vi "NIMS_NS_iir_lpnormconstr.vi"(5 "Function name":string, 6 "Line number":i32, 7 "Number of outputs requested":i32, 8 "error in (no error)":errorcluster, 11 "[A]":variant[](array[variant])) -> (0 "error out":errorcluster, 3 "[funct(A)]":variant[](array[variant]))   [LabVIEW 2017]
uses:
  <vilib>/imath/engines/lvmath/Functions/Error Handling/error.ctl
  <instcachedir>/0/NIMS_RunTimeType_From StrictType (excl LVString)_1019F277F0A747EDBCA0F6C52CA54500.lvgen/NIMS_RunTimeType_From StrictType (excl LVString)_1019F277F0A747EDBCA0F6C52CA54500_000.vi
  <instcachedir>/0/NIMS_Get Scalar_w Error_1987D997E87247DDAC16EA23A5E9E4FC.lvgen/NIMS_Get Scalar_w Error_1987D997E87247DDAC16EA23A5E9E4FC_000.vi
  <instcachedir>/0/NIMS_Complex To Real_BE01396FDE034E8E94CEBBA1E368668D.lvgen/NIMS_Complex To Real_BE01396FDE034E8E94CEBBA1E368668D_000.vi
  <instcachedir>/0/NIMS_Get Any Vector_w Error - Matrix_9FDB8FBE264C42EDBC8FF9BA66C3EF33.lvgen/NIMS_Get Any Vector_w Error - Matrix_9FDB8FBE264C42EDBC8FF9BA66C3EF33_001.vi
  <instcachedir>/0/NIMS_Get Scalar_w Error_1987D997E87247DDAC16EA23A5E9E4FC.lvgen/NIMS_Get Scalar_w Error_1987D997E87247DDAC16EA23A5E9E4FC_003.vi
  <instcachedir>/0/NIMS_RunTimeType_To Numeric_1CBDAFC4EFAD4045A1DE52278D16738D.lvgen/NIMS_RunTimeType_To Numeric_1CBDAFC4EFAD4045A1DE52278D16738D_000.vi
  <vilib>/addons/Digital Filter Design/NI_DigFilter_MathScript.lvlib
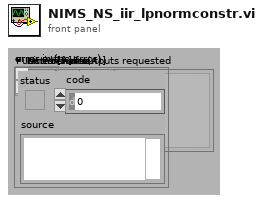
[diagram p1: front panel]
types:
  T1 = typedef "error.ctl" = enum16{"No Error", "Problem", "Input type must not be void", "Incorrect number of parameters", "Function not defined for non-numeric types", "An output variable of the user-defined function is undefined", "Function only defined for character arrays", "Function not defined for boolean, character, or single precision", "Function not defined for complex types", "Not a valid operation", "Inputs must be scalar", "Input matrices are not the same size", "Function only available on RT", "Input matrices must be nonnegative integers of the same type", "Arguments must be non-negative integers less than bitmax", "Number to complement must be less than 2^N", "Bit to get is outside range", "Bit to set is outside range", "Input must be real type ", "At least one parameter must be scalar", "Unable to display plug-in data on RT", "Function not defined for higher dimensional matrices", "Invalid attributes", "Wrong Type of Input Arguments", "Wrong Argument Option", "Invalid file identifier", "Indices must be real positive integers", "The variable is not a matrix data type.", "Number of elements must be the same for indices and values", "You cannot replace elements of a matrix with non-matrix data types.", "Cannot resize a 2D matrix with a linear index", "Unknown variable or symbol", "Indices out of range", "Empty matrix deletion can not be used with two indices", "Number of rows and columns must be the same for indices and values.", "Complex cannot be converted to Boolean", "Char cannot be converted to Boolean", "int64 cannot be converted to Boolean", "uint64 cannot be converted to Boolean", "You cannot convert a Boolean to a character.", "Incompatible input size in 3D surface function", "All rows must have the same number of columns", "Incompatible types", "Invalid matrix dimensions", "Dimension must be 1 or 2", "Base must be an integer between 2 and 36", "Invalid input", "Square matrix required", "Function 'timerstart' must be called before 'timerstop'", "Arguments must be positive real", "Step must not be zero", "Wrong number of input arguments", "Wrong number of output arguments", "Too many index arguments", "Input scalar must be >= 0", "Input scalar must be positive", "Input scalar must not be 0", "Input scalar must be in range [0,1]", "Can't use conditionally defined variable that's undefined", "Input must be a vector", "RT Exec Trace Toolkit not licensed", "Empty vector error", "All elements must be in domain [-1,1]", "All real elements of input vector must be >= 0", "All elements of input vector must be positive", "Values of input vectors are not compatible", "DAQmx not installed", "Input vector must be an increasing vector", "Dereferenced field does not exist within the struct", "A vector or matrix of structures must be indexed before it can be dereferenced", "Lenths of two input vectors are not compatible", "Invalid fieldname", "Empty matrix error", "Cannot use '.' on a type other than Struct", "Unused074", "Data type of the struct's field name is invalid", "Using . to dereference data that is not a struct", "Input struct contains invalid type ", "Size of input matrix is incompatible with input size", "Invalid format specifier", "Could not find field within struct", "Bad permutation array", "Mismatched fieldnames", "ode: User Function could not be opened", "ode: User Function signature does not meet ode requirements", "Unused085", "RunTime: MathScript could not be compiled", "Unknown function", "Only scalars and strings supported", "ode: User Function signature has incorrect number of inputs", "ode:User Function signature has incorrect number of outputs", "Range is too large", "End used without variable", "Function not available (RTE)", "Custom user error", "Arguments must be integers less than bitmax", "Shared library not found", "Header file not found", "Shared library already loaded", "Shared library not loaded", "Shared library function not found", "Shared library string return problem", "Problem calling shared library function", "Problem loading shared library from OS", "Problem parsing shared library header file", "Shared library incompatible types", "Shared library unsupported return type", "Shared library function not exported", "Shared library unsupported input type", "Problem unloading shared library from OS", "Function only available from UI", "Function specified in argument is missing", "An internal error has occurred", "Invalid object", "Invalid property", "Read-only property", "A break command has occurred", "A continue command has occurred", "A return command has occurred", "ode: times parameter invalid", "Function specified in argument has incorrect signature", "Function not found in file", "Reserved keyword cannot be defined as variable", "Reserved keyword cannot be defined as a function or script", "Arguments must be string literals", "Function not supported on this platform", "All columns must have the same number of rows", "Function ignored in RTE warning", "Cannot use : as a parameter that is not a variable", "Output can't be coerced to requested type", "Function not supported on current target", "Variable dependent on an unwired function input", "Unused132", "Unused133", "Unused134", "Unused135", "Unused136", "Unused137", "Unused138", "Unused139", "Global/Persistent must only take constants as arguments.", "Varargin must be last input in the function definition.", "Varargout must be last output in the function definition.", "Invalid output type. Cannot output a cell array of any type other than string.", "Invalid output type. Type is a dynamic struct.", "Invalid output type. Type is a struct that has a field whose type is not known until run-time", "Invalid output type. Type is a struct that has a field which is a plot object.", "MathScript parser DLL missing", "MathScript requires LabVIEW Full", "MathScript license is invalid or missing", "Varargout not supported except in assignments."}
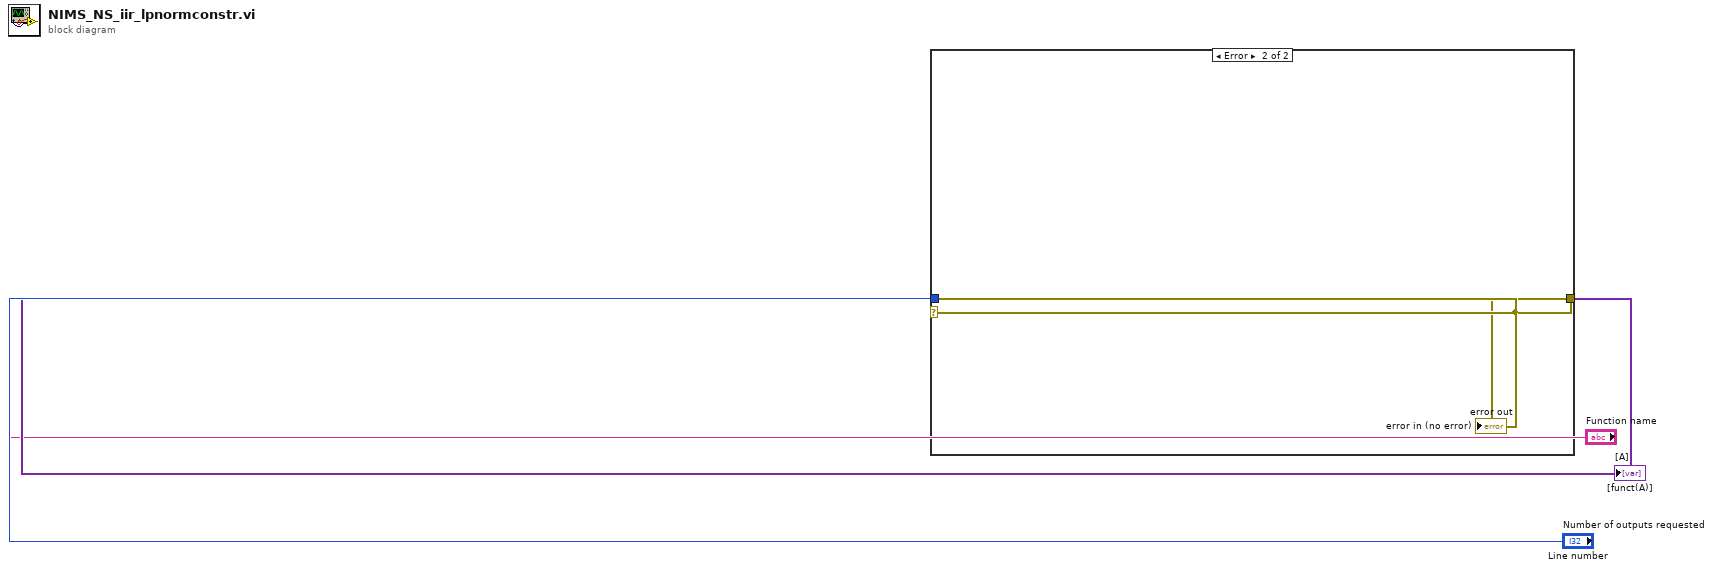
[diagram p0: block diagram]
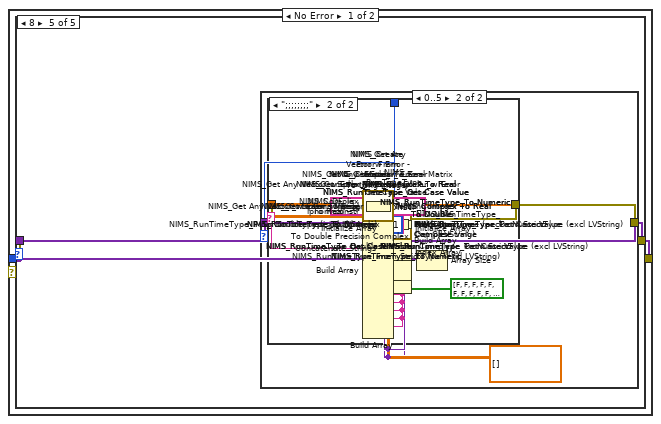
[diagram p2: hidden frame]
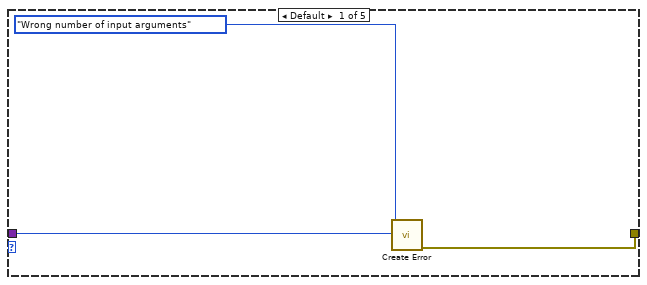
[diagram p3: hidden frame]
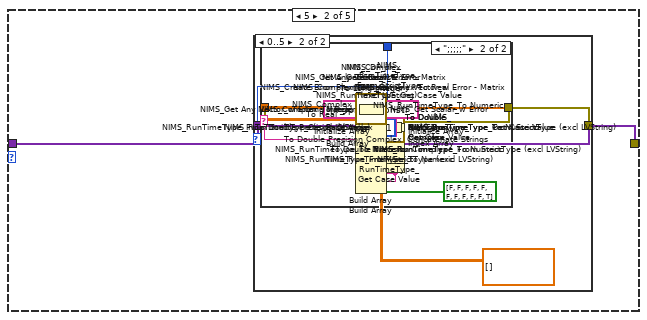
[diagram p4: hidden frame]
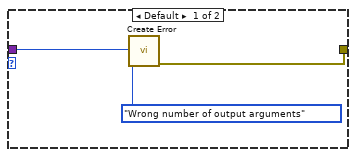
[diagram p5: hidden frame]
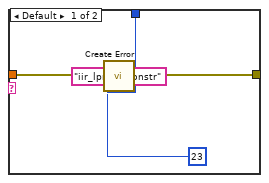
[diagram p6: hidden frame]
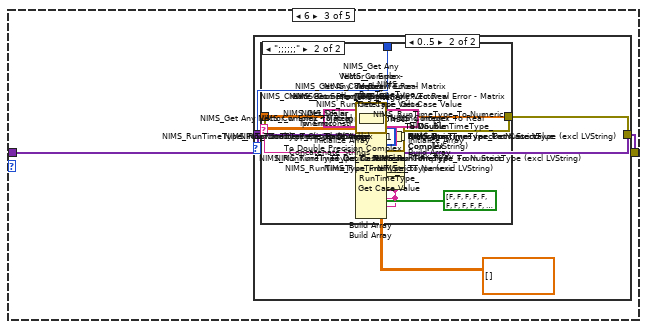
[diagram p7: hidden frame]
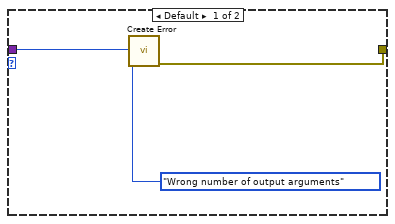
[diagram p8: hidden frame]
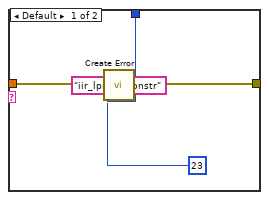
[diagram p9: hidden frame]
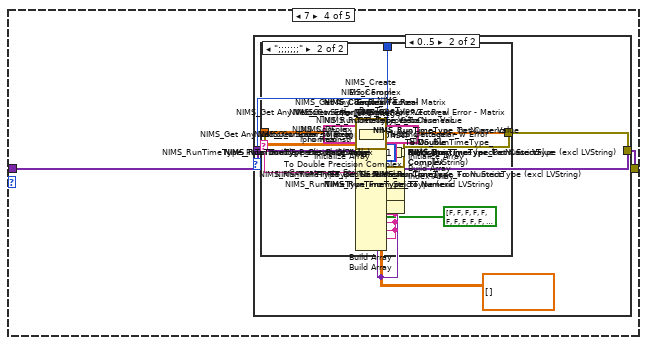
[diagram p10: hidden frame]
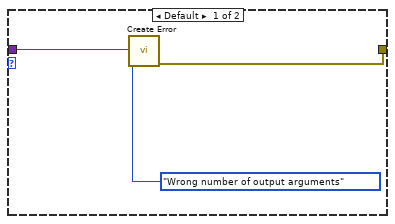
[diagram p11: hidden frame]
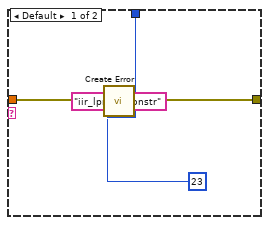
[diagram p12: hidden frame]
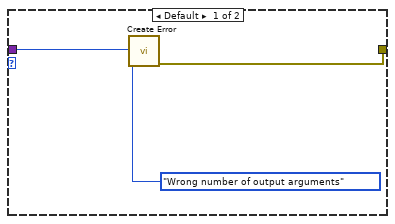
[diagram p13: hidden frame]
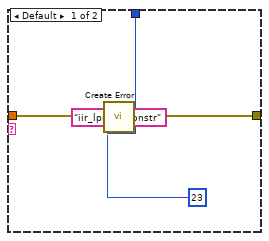
[diagram p14: hidden frame]
diagram:
  n1 = case shown="Error" "error in (no error)" {
    selector: "error in (no error)" -> [_ w516]
    tunnel: [w15 _] -> w4
    tunnel: [w14 w516] -> w3
    tunnel: "error in (no error)" -> [w13 _]
    tunnel: "Number of outputs requested" -> [w12 _]
    tunnel: "[A]" -> [w11 _]
    tunnel: "Function name" -> [w10 _]
    tunnel: "Line number" -> [w9 _]
    frame No Error {
      n2 = Array Size(array=w11) -> (size(s)=w8:i32)
      n3 = case shown="8" w8 {
        tunnel: [_ w27 w137 w256 w384] -> w15
        tunnel: w10 -> [w19 w24 w134 w253 w381]
        tunnel: w9 -> [w20 w25 w135 w254 w382]
        tunnel: w13 -> [w17 w23 w133 w252 w380]
        tunnel: [w16 w22 w132 w251 w379] -> w14
        tunnel: w12 -> [_ w21 w131 w250 w378]
        tunnel: w11 -> [_ w26 w136 w255 w383]
        frame Default {
          n4 = call <vilib>:"Create Error.vi"("Function name"=w19, "error in (no error)"=w17, "Error Enum"=error."Wrong number of input arguments", "Line number"=w20) -> ("error out"=w16:errorcluster)  [unwired: 6 in, 1 out]
        }
        frame 5 {
          n5 = case shown="0..5" w21 {
            tunnel: [_ w33] -> w27
            tunnel: w24 -> [w31 _]
            tunnel: w25 -> [w32 w83]
            tunnel: w23 -> [w29 w81]
            tunnel: [w28 w60] -> w22
            tunnel: w26 -> [_ w84]
            frame Default {
              n6 = call <vilib>:"Create Error.vi"("Function name"=w31, "error in (no error)"=w29, "Error Enum"=error."Wrong number of output arguments", "Line number"=w32) -> ("error out"=w28:errorcluster)  [unwired: 6 in, 1 out]
            }
            frame 0..5 {
              w42 = 1
              w50 = 1
              n7 = Index Array(array=w84) -> (element #1=w80:variant, element #2=w76:variant, element #3=w72:variant, element #4=w68:variant, element #5=w64:variant)  [unwired: 5 in]
              n8 = call <vilib>:"NIMS_RunTimeType_Get Case Value.vi"("Data In"=w64) -> ("Case Value"=w61:string)  [unwired: 9 in, 1 out]
              n9 = call-generic <vilib>:"NIMS_RunTimeType_To Numeric.vi"("DataType"=cdb[][] [], "Variant"=w64) -> ("data"=w62:cdb[][])  [unwired: 1 in]
              n10 = call <vilib>:"NIMS_RunTimeType_Get Case Value.vi"("Data In"=w68) -> ("Case Value"=w65:string)  [unwired: 9 in, 1 out]
              n11 = call-generic <vilib>:"NIMS_RunTimeType_To Numeric.vi"("DataType"=cdb[][] [], "Variant"=w68) -> ("data"=w66:cdb[][])  [unwired: 1 in]
              n12 = call <vilib>:"NIMS_RunTimeType_Get Case Value.vi"("Data In"=w72) -> ("Case Value"=w69:string)  [unwired: 9 in, 1 out]
              n13 = call-generic <vilib>:"NIMS_RunTimeType_To Numeric.vi"("DataType"=cdb[][] [], "Variant"=w72) -> ("data"=w70:cdb[][])  [unwired: 1 in]
              n14 = call <vilib>:"NIMS_RunTimeType_Get Case Value.vi"("Data In"=w76) -> ("Case Value"=w73:string)  [unwired: 9 in, 1 out]
              n15 = call-generic <vilib>:"NIMS_RunTimeType_To Numeric.vi"("DataType"=cdb[][] [], "Variant"=w76) -> ("data"=w74:cdb[][])  [unwired: 1 in]
              n16 = call <vilib>:"NIMS_RunTimeType_Get Case Value.vi"("Data In"=w80) -> ("Case Value"=w77:string)  [unwired: 9 in, 1 out]
              n17 = call-generic <vilib>:"NIMS_RunTimeType_To Numeric.vi"("DataType"=cdb[][] [], "Variant"=w80) -> ("data"=w78:cdb[][])  [unwired: 1 in]
              n18 = Concatenate Strings(w77, w73, w69, w65, w61) -> (w82:string)
              n19 = case shown="\";;;;;\"" w82 {
                tunnel: w81 -> [w86 w99]
                tunnel: [_ w94] -> w59
                tunnel: [_ w93] -> w55
                tunnel: [_ w92] -> w51
                tunnel: [_ w91] -> w46
                tunnel: [_ w90] -> w43
                tunnel: [w85 w95] -> w60
                tunnel: w78 -> [_ w129]
                tunnel: w74 -> [_ w125]
                tunnel: w70 -> [_ w121]
                tunnel: w66 -> [_ w118]
                tunnel: w62 -> [_ w115]
                tunnel: w83 -> [w89 w102]
                frame Default {
                  n20 = call <vilib>:"Create Error.vi"("Function name"="iir_lpnormconstr", "error in (no error)"=w86, "Error Enum"=23, "Line number"=w89) -> ("error out"=w85:errorcluster)  [unwired: 6 in, 1 out]
                }
                frame ";;;;;" {
                  w97 = "iir_lpnormconstr"
                  n21 = call-generic <vilib>:"NIMS_Complex To Real.vi"("A"=w115) -> ("Error Enum"=w105:T1, "Real(A)"=w114:dbl[][])  [unwired: 8 in, 1 out]
                  n22 = call-generic <vilib>:"NIMS_Get Any Vector_w Error - Matrix.vi"("A"=w114) -> ("Error Enum"=w104:T1, "Vector"=w116:dbl[])  [unwired: 8 in, 1 out]
                  n23 = call-generic <vilib>:"NIMS_Complex To Real.vi"("A"=w118) -> ("Error Enum"=w107:T1, "Real(A)"=w117:dbl[][])  [unwired: 8 in, 1 out]
                  n24 = call-generic <vilib>:"NIMS_Get Any Vector_w Error - Matrix.vi"("A"=w117) -> ("Error Enum"=w106:T1, "Vector"=w119:dbl[])  [unwired: 8 in, 1 out]
                  n25 = call-generic <vilib>:"NIMS_Complex To Real.vi"("A"=w121) -> ("Error Enum"=w109:T1, "Real(A)"=w120:dbl[][])  [unwired: 8 in, 1 out]
                  n26 = call-generic <vilib>:"NIMS_Get Any Vector_w Error - Matrix.vi"("A"=w120) -> ("Error Enum"=w108:T1, "Vector"=w122:dbl[])  [unwired: 8 in, 1 out]
                  n27 = call-generic <vilib>:"NIMS_Complex To Real.vi"("A"=w125) -> ("Error Enum"=w111:T1, "Real(A)"=w124:dbl[][])  [unwired: 8 in, 1 out]
                  n28 = To Long Integer(number=w124) -> (32bit integer=w123:i32[][])
                  n29 = call-generic <vilib>:"NIMS_Get Scalar_w Error.vi"("A"=w123) -> ("Error Enum"=w110:T1, "Scalar"=w126:i32)  [unwired: 8 in, 1 out]
                  n30 = call-generic <vilib>:"NIMS_Complex To Real.vi"("A"=w129) -> ("Error Enum"=w113:T1, "Real(A)"=w128:dbl[][])  [unwired: 8 in, 1 out]
                  n31 = To Long Integer(number=w128) -> (32bit integer=w127:i32[][])
                  n32 = call-generic <vilib>:"NIMS_Get Scalar_w Error.vi"("A"=w127) -> ("Error Enum"=w112:T1, "Scalar"=w130:i32)  [unwired: 8 in, 1 out]
                  n33 = call <vilib>:"NIMS_DF_iir_lpnormconstr.vi"("n"=w130, "e"=w119, "d"=w126, "f"=w122, "mag"=w116) -> ("b"=w94:dbl[], "a"=w93:dbl[], "err"=w92:dbl, "SOS"=w91:dbl[][], "error"=w103:i32, "gain"=w90:dbl)  [unwired: 5 in]
                  n34 = Build Array(w97, w97, w97, w97, w97, w97, w97, w97, w97, w97, "iir_lpnormconstr") -> (w100:string[])
                  n35 = Build Array(w113, w112, w111, w110, w109, w108, w107, w106, w105, w104, w103) -> (w101:i32[])
                  n36 = call <vilib>:"NIMS_Create Error From Enums.vi"("Error Code"=bool[] [FALSE, FALSE, FALSE, FALSE, FALSE, FALSE, FALSE, FALSE, FALSE, FALSE, TRUE], "error in (no error)"=w99, "Line no"=w102, "Error Enums"=w101, "Function names"=w100) -> ("error out"=w95:errorcluster)  [unwired: 6 in]
                }
              }
              n37 = To Double Precision Complex(1:w46) -> (0:w45:cdb[][])
              n38 = call-generic <vilib>:"NIMS_RunTimeType_From StrictType (excl LVString).vi"("Plug-In Name"="", "Data In"=w45) -> ("Data Out"=w35:variant)  [unwired: 2 in]
              n39 = Initialize Array(w43, w42, w42) -> (w41:dbl[][])
              n40 = To Double Precision Complex(1:w41) -> (0:w40:cdb[][])
              n41 = call-generic <vilib>:"NIMS_RunTimeType_From StrictType (excl LVString).vi"("Plug-In Name"="", "Data In"=w40) -> ("Data Out"=w34:variant)  [unwired: 2 in]
              n42 = Initialize Array(w51, w50, w50) -> (w49:dbl[][])
              n43 = To Double Precision Complex(1:w49) -> (0:w48:cdb[][])
              n44 = call-generic <vilib>:"NIMS_RunTimeType_From StrictType (excl LVString).vi"("Plug-In Name"="", "Data In"=w48) -> ("Data Out"=w36:variant)  [unwired: 2 in]
              n45 = Build Array(w55) -> (w54:dbl[][])
              n46 = To Double Precision Complex(1:w54) -> (0:w53:cdb[][])
              n47 = call-generic <vilib>:"NIMS_RunTimeType_From StrictType (excl LVString).vi"("Plug-In Name"="", "Data In"=w53) -> ("Data Out"=w37:variant)  [unwired: 2 in]
              n48 = Build Array(w59) -> (w58:dbl[][])
              n49 = To Double Precision Complex(1:w58) -> (0:w57:cdb[][])
              n50 = call-generic <vilib>:"NIMS_RunTimeType_From StrictType (excl LVString).vi"("Plug-In Name"="", "Data In"=w57) -> ("Data Out"=w38:variant)  [unwired: 2 in]
              n51 = Build Array(w38, w37, w36, w35, w34) -> (w33:variant[])
            }
          }
        }
        frame 6 {
          n52 = case shown="0..5" w131 {
            tunnel: [_ w143] -> w137
            tunnel: w134 -> [w141 _]
            tunnel: w135 -> [w142 w197]
            tunnel: w133 -> [w139 w195]
            tunnel: [w138 w170] -> w132
            tunnel: w136 -> [_ w198]
            frame Default {
              n53 = call <vilib>:"Create Error.vi"("Function name"=w141, "error in (no error)"=w139, "Error Enum"=error."Wrong number of output arguments", "Line number"=w142) -> ("error out"=w138:errorcluster)  [unwired: 6 in, 1 out]
            }
            frame 0..5 {
              w152 = 1
              w160 = 1
              n54 = Index Array(array=w198) -> (element #1=w194:variant, element #2=w190:variant, element #3=w186:variant, element #4=w182:variant, element #5=w178:variant, element #6=w174:variant)  [unwired: 6 in]
              n55 = call <vilib>:"NIMS_RunTimeType_Get Case Value.vi"("Data In"=w174) -> ("Case Value"=w171:string)  [unwired: 9 in, 1 out]
              n56 = call-generic <vilib>:"NIMS_RunTimeType_To Numeric.vi"("DataType"=cdb[][] [], "Variant"=w174) -> ("data"=w172:cdb[][])  [unwired: 1 in]
              n57 = call <vilib>:"NIMS_RunTimeType_Get Case Value.vi"("Data In"=w178) -> ("Case Value"=w175:string)  [unwired: 9 in, 1 out]
              n58 = call-generic <vilib>:"NIMS_RunTimeType_To Numeric.vi"("DataType"=cdb[][] [], "Variant"=w178) -> ("data"=w176:cdb[][])  [unwired: 1 in]
              n59 = call <vilib>:"NIMS_RunTimeType_Get Case Value.vi"("Data In"=w182) -> ("Case Value"=w179:string)  [unwired: 9 in, 1 out]
              n60 = call-generic <vilib>:"NIMS_RunTimeType_To Numeric.vi"("DataType"=cdb[][] [], "Variant"=w182) -> ("data"=w180:cdb[][])  [unwired: 1 in]
              n61 = call <vilib>:"NIMS_RunTimeType_Get Case Value.vi"("Data In"=w186) -> ("Case Value"=w183:string)  [unwired: 9 in, 1 out]
              n62 = call-generic <vilib>:"NIMS_RunTimeType_To Numeric.vi"("DataType"=cdb[][] [], "Variant"=w186) -> ("data"=w184:cdb[][])  [unwired: 1 in]
              n63 = call <vilib>:"NIMS_RunTimeType_Get Case Value.vi"("Data In"=w190) -> ("Case Value"=w187:string)  [unwired: 9 in, 1 out]
              n64 = call-generic <vilib>:"NIMS_RunTimeType_To Numeric.vi"("DataType"=cdb[][] [], "Variant"=w190) -> ("data"=w188:cdb[][])  [unwired: 1 in]
              n65 = call <vilib>:"NIMS_RunTimeType_Get Case Value.vi"("Data In"=w194) -> ("Case Value"=w191:string)  [unwired: 9 in, 1 out]
              n66 = call-generic <vilib>:"NIMS_RunTimeType_To Numeric.vi"("DataType"=cdb[][] [], "Variant"=w194) -> ("data"=w192:cdb[][])  [unwired: 1 in]
              n67 = Concatenate Strings(w191, w187, w183, w179, w175, w171) -> (w196:string)
              n68 = case shown="\";;;;;;\"" w196 {
                tunnel: w195 -> [w200 w213]
                tunnel: [_ w208] -> w169
                tunnel: [_ w207] -> w165
                tunnel: [_ w206] -> w161
                tunnel: [_ w205] -> w156
                tunnel: [_ w204] -> w153
                tunnel: [w199 w209] -> w170
                tunnel: w192 -> [_ w248]
                tunnel: w188 -> [_ w244]
                tunnel: w184 -> [_ w240]
                tunnel: w180 -> [_ w237]
                tunnel: w176 -> [_ w234]
                tunnel: w172 -> [_ w231]
                tunnel: w197 -> [w203 w216]
                frame Default {
                  n69 = call <vilib>:"Create Error.vi"("Function name"="iir_lpnormconstr", "error in (no error)"=w200, "Error Enum"=23, "Line number"=w203) -> ("error out"=w199:errorcluster)  [unwired: 6 in, 1 out]
                }
                frame ";;;;;;" {
                  w211 = "iir_lpnormconstr"
                  n70 = call-generic <vilib>:"NIMS_Complex To Real.vi"("A"=w231) -> ("Error Enum"=w219:T1, "Real(A)"=w230:dbl[][])  [unwired: 8 in, 1 out]
                  n71 = call-generic <vilib>:"NIMS_Get Any Vector_w Error - Matrix.vi"("A"=w230) -> ("Error Enum"=w218:T1, "Vector"=w232:dbl[])  [unwired: 8 in, 1 out]
                  n72 = call-generic <vilib>:"NIMS_Complex To Real.vi"("A"=w234) -> ("Error Enum"=w221:T1, "Real(A)"=w233:dbl[][])  [unwired: 8 in, 1 out]
                  n73 = call-generic <vilib>:"NIMS_Get Any Vector_w Error - Matrix.vi"("A"=w233) -> ("Error Enum"=w220:T1, "Vector"=w235:dbl[])  [unwired: 8 in, 1 out]
                  n74 = call-generic <vilib>:"NIMS_Complex To Real.vi"("A"=w237) -> ("Error Enum"=w223:T1, "Real(A)"=w236:dbl[][])  [unwired: 8 in, 1 out]
                  n75 = call-generic <vilib>:"NIMS_Get Any Vector_w Error - Matrix.vi"("A"=w236) -> ("Error Enum"=w222:T1, "Vector"=w238:dbl[])  [unwired: 8 in, 1 out]
                  n76 = call-generic <vilib>:"NIMS_Complex To Real.vi"("A"=w240) -> ("Error Enum"=w225:T1, "Real(A)"=w239:dbl[][])  [unwired: 8 in, 1 out]
                  n77 = call-generic <vilib>:"NIMS_Get Any Vector_w Error - Matrix.vi"("A"=w239) -> ("Error Enum"=w224:T1, "Vector"=w241:dbl[])  [unwired: 8 in, 1 out]
                  n78 = call-generic <vilib>:"NIMS_Complex To Real.vi"("A"=w244) -> ("Error Enum"=w227:T1, "Real(A)"=w243:dbl[][])  [unwired: 8 in, 1 out]
                  n79 = To Long Integer(number=w243) -> (32bit integer=w242:i32[][])
                  n80 = call-generic <vilib>:"NIMS_Get Scalar_w Error.vi"("A"=w242) -> ("Error Enum"=w226:T1, "Scalar"=w245:i32)  [unwired: 8 in, 1 out]
                  n81 = call-generic <vilib>:"NIMS_Complex To Real.vi"("A"=w248) -> ("Error Enum"=w229:T1, "Real(A)"=w247:dbl[][])  [unwired: 8 in, 1 out]
                  n82 = To Long Integer(number=w247) -> (32bit integer=w246:i32[][])
                  n83 = call-generic <vilib>:"NIMS_Get Scalar_w Error.vi"("A"=w246) -> ("Error Enum"=w228:T1, "Scalar"=w249:i32)  [unwired: 8 in, 1 out]
                  n84 = call <vilib>:"NIMS_DF_iir_lpnormconstr.vi"("n"=w249, "e"=w238, "w"=w232, "d"=w245, "f"=w241, "mag"=w235) -> ("b"=w208:dbl[], "a"=w207:dbl[], "err"=w206:dbl, "SOS"=w205:dbl[][], "error"=w217:i32, "gain"=w204:dbl)  [unwired: 4 in]
                  n85 = Build Array(w211, w211, w211, w211, w211, w211, w211, w211, w211, w211, w211, w211, "iir_lpnormconstr") -> (w214:string[])
                  n86 = Build Array(w229, w228, w227, w226, w225, w224, w223, w222, w221, w220, w219, w218, w217) -> (w215:i32[])
                  n87 = call <vilib>:"NIMS_Create Error From Enums.vi"("Error Code"=bool[] [FALSE, FALSE, FALSE, FALSE, FALSE, FALSE, FALSE, FALSE, FALSE, FALSE, FALSE, FALSE, TRUE], "error in (no error)"=w213, "Line no"=w216, "Error Enums"=w215, "Function names"=w214) -> ("error out"=w209:errorcluster)  [unwired: 6 in]
                }
              }
              n88 = To Double Precision Complex(1:w156) -> (0:w155:cdb[][])
              n89 = call-generic <vilib>:"NIMS_RunTimeType_From StrictType (excl LVString).vi"("Plug-In Name"="", "Data In"=w155) -> ("Data Out"=w145:variant)  [unwired: 2 in]
              n90 = Initialize Array(w153, w152, w152) -> (w151:dbl[][])
              n91 = To Double Precision Complex(1:w151) -> (0:w150:cdb[][])
              n92 = call-generic <vilib>:"NIMS_RunTimeType_From StrictType (excl LVString).vi"("Plug-In Name"="", "Data In"=w150) -> ("Data Out"=w144:variant)  [unwired: 2 in]
              n93 = Initialize Array(w161, w160, w160) -> (w159:dbl[][])
              n94 = To Double Precision Complex(1:w159) -> (0:w158:cdb[][])
              n95 = call-generic <vilib>:"NIMS_RunTimeType_From StrictType (excl LVString).vi"("Plug-In Name"="", "Data In"=w158) -> ("Data Out"=w146:variant)  [unwired: 2 in]
              n96 = Build Array(w165) -> (w164:dbl[][])
              n97 = To Double Precision Complex(1:w164) -> (0:w163:cdb[][])
              n98 = call-generic <vilib>:"NIMS_RunTimeType_From StrictType (excl LVString).vi"("Plug-In Name"="", "Data In"=w163) -> ("Data Out"=w147:variant)  [unwired: 2 in]
              n99 = Build Array(w169) -> (w168:dbl[][])
              n100 = To Double Precision Complex(1:w168) -> (0:w167:cdb[][])
              n101 = call-generic <vilib>:"NIMS_RunTimeType_From StrictType (excl LVString).vi"("Plug-In Name"="", "Data In"=w167) -> ("Data Out"=w148:variant)  [unwired: 2 in]
              n102 = Build Array(w148, w147, w146, w145, w144) -> (w143:variant[])
            }
          }
        }
        frame 7 {
          n103 = case shown="0..5" w250 {
            tunnel: [_ w262] -> w256
            tunnel: w253 -> [w260 _]
            tunnel: w254 -> [w261 w320]
            tunnel: w252 -> [w258 w318]
            tunnel: [w257 w289] -> w251
            tunnel: w255 -> [_ w321]
            frame Default {
              n104 = call <vilib>:"Create Error.vi"("Function name"=w260, "error in (no error)"=w258, "Error Enum"=error."Wrong number of output arguments", "Line number"=w261) -> ("error out"=w257:errorcluster)  [unwired: 6 in, 1 out]
            }
            frame 0..5 {
              w271 = 1
              w279 = 1
              n105 = Index Array(array=w321) -> (element #1=w317:variant, element #2=w313:variant, element #3=w309:variant, element #4=w305:variant, element #5=w301:variant, element #6=w297:variant, element #7=w293:variant)  [unwired: 7 in]
              n106 = call <vilib>:"NIMS_RunTimeType_Get Case Value.vi"("Data In"=w293) -> ("Case Value"=w290:string)  [unwired: 9 in, 1 out]
              n107 = call-generic <vilib>:"NIMS_RunTimeType_To Numeric.vi"("DataType"=cdb[][] [], "Variant"=w293) -> ("data"=w291:cdb[][])  [unwired: 1 in]
              n108 = call <vilib>:"NIMS_RunTimeType_Get Case Value.vi"("Data In"=w297) -> ("Case Value"=w294:string)  [unwired: 9 in, 1 out]
              n109 = call-generic <vilib>:"NIMS_RunTimeType_To Numeric.vi"("DataType"=cdb[][] [], "Variant"=w297) -> ("data"=w295:cdb[][])  [unwired: 1 in]
              n110 = call <vilib>:"NIMS_RunTimeType_Get Case Value.vi"("Data In"=w301) -> ("Case Value"=w298:string)  [unwired: 9 in, 1 out]
              n111 = call-generic <vilib>:"NIMS_RunTimeType_To Numeric.vi"("DataType"=cdb[][] [], "Variant"=w301) -> ("data"=w299:cdb[][])  [unwired: 1 in]
              n112 = call <vilib>:"NIMS_RunTimeType_Get Case Value.vi"("Data In"=w305) -> ("Case Value"=w302:string)  [unwired: 9 in, 1 out]
              n113 = call-generic <vilib>:"NIMS_RunTimeType_To Numeric.vi"("DataType"=cdb[][] [], "Variant"=w305) -> ("data"=w303:cdb[][])  [unwired: 1 in]
              n114 = call <vilib>:"NIMS_RunTimeType_Get Case Value.vi"("Data In"=w309) -> ("Case Value"=w306:string)  [unwired: 9 in, 1 out]
              n115 = call-generic <vilib>:"NIMS_RunTimeType_To Numeric.vi"("DataType"=cdb[][] [], "Variant"=w309) -> ("data"=w307:cdb[][])  [unwired: 1 in]
              n116 = call <vilib>:"NIMS_RunTimeType_Get Case Value.vi"("Data In"=w313) -> ("Case Value"=w310:string)  [unwired: 9 in, 1 out]
              n117 = call-generic <vilib>:"NIMS_RunTimeType_To Numeric.vi"("DataType"=cdb[][] [], "Variant"=w313) -> ("data"=w311:cdb[][])  [unwired: 1 in]
              n118 = call <vilib>:"NIMS_RunTimeType_Get Case Value.vi"("Data In"=w317) -> ("Case Value"=w314:string)  [unwired: 9 in, 1 out]
              n119 = call-generic <vilib>:"NIMS_RunTimeType_To Numeric.vi"("DataType"=cdb[][] [], "Variant"=w317) -> ("data"=w315:cdb[][])  [unwired: 1 in]
              n120 = Concatenate Strings(w314, w310, w306, w302, w298, w294, w290) -> (w319:string)
              n121 = case shown="\";;;;;;;\"" w319 {
                tunnel: w318 -> [w323 w336]
                tunnel: [_ w331] -> w288
                tunnel: [_ w330] -> w284
                tunnel: [_ w329] -> w280
                tunnel: [_ w328] -> w275
                tunnel: [_ w327] -> w272
                tunnel: [w322 w332] -> w289
                tunnel: w315 -> [_ w376]
                tunnel: w311 -> [_ w372]
                tunnel: w307 -> [_ w368]
                tunnel: w303 -> [_ w365]
                tunnel: w299 -> [_ w362]
                tunnel: w295 -> [_ w359]
                tunnel: w291 -> [_ w356]
                tunnel: w320 -> [w326 w339]
                frame Default {
                  n122 = call <vilib>:"Create Error.vi"("Function name"="iir_lpnormconstr", "error in (no error)"=w323, "Error Enum"=23, "Line number"=w326) -> ("error out"=w322:errorcluster)  [unwired: 6 in, 1 out]
                }
                frame ";;;;;;;" {
                  w334 = "iir_lpnormconstr"
                  n123 = call-generic <vilib>:"NIMS_Complex To Real.vi"("A"=w356) -> ("Error Enum"=w342:T1, "Real(A)"=w355:dbl[][])  [unwired: 8 in, 1 out]
                  n124 = call-generic <vilib>:"NIMS_Get Scalar_w Error.vi"("A"=w355) -> ("Error Enum"=w341:T1, "Scalar"=w357:dbl)  [unwired: 8 in, 1 out]
                  n125 = call-generic <vilib>:"NIMS_Complex To Real.vi"("A"=w359) -> ("Error Enum"=w344:T1, "Real(A)"=w358:dbl[][])  [unwired: 8 in, 1 out]
                  n126 = call-generic <vilib>:"NIMS_Get Any Vector_w Error - Matrix.vi"("A"=w358) -> ("Error Enum"=w343:T1, "Vector"=w360:dbl[])  [unwired: 8 in, 1 out]
                  n127 = call-generic <vilib>:"NIMS_Complex To Real.vi"("A"=w362) -> ("Error Enum"=w346:T1, "Real(A)"=w361:dbl[][])  [unwired: 8 in, 1 out]
                  n128 = call-generic <vilib>:"NIMS_Get Any Vector_w Error - Matrix.vi"("A"=w361) -> ("Error Enum"=w345:T1, "Vector"=w363:dbl[])  [unwired: 8 in, 1 out]
                  n129 = call-generic <vilib>:"NIMS_Complex To Real.vi"("A"=w365) -> ("Error Enum"=w348:T1, "Real(A)"=w364:dbl[][])  [unwired: 8 in, 1 out]
                  n130 = call-generic <vilib>:"NIMS_Get Any Vector_w Error - Matrix.vi"("A"=w364) -> ("Error Enum"=w347:T1, "Vector"=w366:dbl[])  [unwired: 8 in, 1 out]
                  n131 = call-generic <vilib>:"NIMS_Complex To Real.vi"("A"=w368) -> ("Error Enum"=w350:T1, "Real(A)"=w367:dbl[][])  [unwired: 8 in, 1 out]
                  n132 = call-generic <vilib>:"NIMS_Get Any Vector_w Error - Matrix.vi"("A"=w367) -> ("Error Enum"=w349:T1, "Vector"=w369:dbl[])  [unwired: 8 in, 1 out]
                  n133 = call-generic <vilib>:"NIMS_Complex To Real.vi"("A"=w372) -> ("Error Enum"=w352:T1, "Real(A)"=w371:dbl[][])  [unwired: 8 in, 1 out]
                  n134 = To Long Integer(number=w371) -> (32bit integer=w370:i32[][])
                  n135 = call-generic <vilib>:"NIMS_Get Scalar_w Error.vi"("A"=w370) -> ("Error Enum"=w351:T1, "Scalar"=w373:i32)  [unwired: 8 in, 1 out]
                  n136 = call-generic <vilib>:"NIMS_Complex To Real.vi"("A"=w376) -> ("Error Enum"=w354:T1, "Real(A)"=w375:dbl[][])  [unwired: 8 in, 1 out]
                  n137 = To Long Integer(number=w375) -> (32bit integer=w374:i32[][])
                  n138 = call-generic <vilib>:"NIMS_Get Scalar_w Error.vi"("A"=w374) -> ("Error Enum"=w353:T1, "Scalar"=w377:i32)  [unwired: 8 in, 1 out]
                  n139 = call <vilib>:"NIMS_DF_iir_lpnormconstr.vi"("n"=w377, "e"=w366, "w"=w360, "d"=w373, "f"=w369, "mag"=w363, "r"=w357) -> ("b"=w331:dbl[], "a"=w330:dbl[], "err"=w329:dbl, "SOS"=w328:dbl[][], "error"=w340:i32, "gain"=w327:dbl)  [unwired: 3 in]
                  n140 = Build Array(w334, w334, w334, w334, w334, w334, w334, w334, w334, w334, w334, w334, w334, w334, "iir_lpnormconstr") -> (w337:string[])
                  n141 = Build Array(w354, w353, w352, w351, w350, w349, w348, w347, w346, w345, w344, w343, w342, w341, w340) -> (w338:i32[])
                  n142 = call <vilib>:"NIMS_Create Error From Enums.vi"("Error Code"=bool[] [FALSE, FALSE, FALSE, FALSE, FALSE, FALSE, FALSE, FALSE, FALSE, FALSE, FALSE, FALSE, FALSE, FALSE, TRUE], "error in (no error)"=w336, "Line no"=w339, "Error Enums"=w338, "Function names"=w337) -> ("error out"=w332:errorcluster)  [unwired: 6 in]
                }
              }
              n143 = To Double Precision Complex(1:w275) -> (0:w274:cdb[][])
              n144 = call-generic <vilib>:"NIMS_RunTimeType_From StrictType (excl LVString).vi"("Plug-In Name"="", "Data In"=w274) -> ("Data Out"=w264:variant)  [unwired: 2 in]
              n145 = Initialize Array(w272, w271, w271) -> (w270:dbl[][])
              n146 = To Double Precision Complex(1:w270) -> (0:w269:cdb[][])
              n147 = call-generic <vilib>:"NIMS_RunTimeType_From StrictType (excl LVString).vi"("Plug-In Name"="", "Data In"=w269) -> ("Data Out"=w263:variant)  [unwired: 2 in]
              n148 = Initialize Array(w280, w279, w279) -> (w278:dbl[][])
              n149 = To Double Precision Complex(1:w278) -> (0:w277:cdb[][])
              n150 = call-generic <vilib>:"NIMS_RunTimeType_From StrictType (excl LVString).vi"("Plug-In Name"="", "Data In"=w277) -> ("Data Out"=w265:variant)  [unwired: 2 in]
              n151 = Build Array(w284) -> (w283:dbl[][])
              n152 = To Double Precision Complex(1:w283) -> (0:w282:cdb[][])
              n153 = call-generic <vilib>:"NIMS_RunTimeType_From StrictType (excl LVString).vi"("Plug-In Name"="", "Data In"=w282) -> ("Data Out"=w266:variant)  [unwired: 2 in]
              n154 = Build Array(w288) -> (w287:dbl[][])
              n155 = To Double Precision Complex(1:w287) -> (0:w286:cdb[][])
              n156 = call-generic <vilib>:"NIMS_RunTimeType_From StrictType (excl LVString).vi"("Plug-In Name"="", "Data In"=w286) -> ("Data Out"=w267:variant)  [unwired: 2 in]
              n157 = Build Array(w267, w266, w265, w264, w263) -> (w262:variant[])
            }
          }
        }
        frame 8 {
          n158 = case shown="0..5" w378 {
            tunnel: [_ w390] -> w384
            tunnel: w381 -> [w388 _]
            tunnel: w382 -> [w389 w452]
            tunnel: w380 -> [w386 w450]
            tunnel: [w385 w417] -> w379
            tunnel: w383 -> [_ w453]
            frame Default {
              n159 = call <vilib>:"Create Error.vi"("Function name"=w388, "error in (no error)"=w386, "Error Enum"=error."Wrong number of output arguments", "Line number"=w389) -> ("error out"=w385:errorcluster)  [unwired: 6 in, 1 out]
            }
            frame 0..5 {
              w399 = 1
              w407 = 1
              n160 = Index Array(array=w453) -> (element #1=w449:variant, element #2=w445:variant, element #3=w441:variant, element #4=w437:variant, element #5=w433:variant, element #6=w429:variant, element #7=w425:variant, element #8=w421:variant)  [unwired: 8 in]
              n161 = call <vilib>:"NIMS_RunTimeType_Get Case Value.vi"("Data In"=w421) -> ("Case Value"=w418:string)  [unwired: 9 in, 1 out]
              n162 = call-generic <vilib>:"NIMS_RunTimeType_To Numeric.vi"("DataType"=cdb[][] [], "Variant"=w421) -> ("data"=w419:cdb[][])  [unwired: 1 in]
              n163 = call <vilib>:"NIMS_RunTimeType_Get Case Value.vi"("Data In"=w425) -> ("Case Value"=w422:string)  [unwired: 9 in, 1 out]
              n164 = call-generic <vilib>:"NIMS_RunTimeType_To Numeric.vi"("DataType"=cdb[][] [], "Variant"=w425) -> ("data"=w423:cdb[][])  [unwired: 1 in]
              n165 = call <vilib>:"NIMS_RunTimeType_Get Case Value.vi"("Data In"=w429) -> ("Case Value"=w426:string)  [unwired: 9 in, 1 out]
              n166 = call-generic <vilib>:"NIMS_RunTimeType_To Numeric.vi"("DataType"=cdb[][] [], "Variant"=w429) -> ("data"=w427:cdb[][])  [unwired: 1 in]
              n167 = call <vilib>:"NIMS_RunTimeType_Get Case Value.vi"("Data In"=w433) -> ("Case Value"=w430:string)  [unwired: 9 in, 1 out]
              n168 = call-generic <vilib>:"NIMS_RunTimeType_To Numeric.vi"("DataType"=cdb[][] [], "Variant"=w433) -> ("data"=w431:cdb[][])  [unwired: 1 in]
              n169 = call <vilib>:"NIMS_RunTimeType_Get Case Value.vi"("Data In"=w437) -> ("Case Value"=w434:string)  [unwired: 9 in, 1 out]
              n170 = call-generic <vilib>:"NIMS_RunTimeType_To Numeric.vi"("DataType"=cdb[][] [], "Variant"=w437) -> ("data"=w435:cdb[][])  [unwired: 1 in]
              n171 = call <vilib>:"NIMS_RunTimeType_Get Case Value.vi"("Data In"=w441) -> ("Case Value"=w438:string)  [unwired: 9 in, 1 out]
              n172 = call-generic <vilib>:"NIMS_RunTimeType_To Numeric.vi"("DataType"=cdb[][] [], "Variant"=w441) -> ("data"=w439:cdb[][])  [unwired: 1 in]
              n173 = call <vilib>:"NIMS_RunTimeType_Get Case Value.vi"("Data In"=w445) -> ("Case Value"=w442:string)  [unwired: 9 in, 1 out]
              n174 = call-generic <vilib>:"NIMS_RunTimeType_To Numeric.vi"("DataType"=cdb[][] [], "Variant"=w445) -> ("data"=w443:cdb[][])  [unwired: 1 in]
              n175 = call <vilib>:"NIMS_RunTimeType_Get Case Value.vi"("Data In"=w449) -> ("Case Value"=w446:string)  [unwired: 9 in, 1 out]
              n176 = call-generic <vilib>:"NIMS_RunTimeType_To Numeric.vi"("DataType"=cdb[][] [], "Variant"=w449) -> ("data"=w447:cdb[][])  [unwired: 1 in]
              n177 = Concatenate Strings(w446, w442, w438, w434, w430, w426, w422, w418) -> (w451:string)
              n178 = case shown="\";;;;;;;;\"" w451 {
                tunnel: w450 -> [w455 w468]
                tunnel: [_ w463] -> w416
                tunnel: [_ w462] -> w412
                tunnel: [_ w461] -> w408
                tunnel: [_ w460] -> w403
                tunnel: [_ w459] -> w400
                tunnel: [w454 w464] -> w417
                tunnel: w447 -> [_ w514]
                tunnel: w443 -> [_ w510]
                tunnel: w439 -> [_ w506]
                tunnel: w435 -> [_ w503]
                tunnel: w431 -> [_ w500]
                tunnel: w427 -> [_ w497]
                tunnel: w423 -> [_ w494]
                tunnel: w419 -> [_ w491]
                tunnel: w452 -> [w458 w471]
                frame Default {
                  n179 = call <vilib>:"Create Error.vi"("Function name"="iir_lpnormconstr", "error in (no error)"=w455, "Error Enum"=23, "Line number"=w458) -> ("error out"=w454:errorcluster)  [unwired: 6 in, 1 out]
                }
                frame ";;;;;;;;" {
                  w466 = "iir_lpnormconstr"
                  n180 = call-generic <vilib>:"NIMS_Complex To Real.vi"("A"=w491) -> ("Error Enum"=w474:T1, "Real(A)"=w490:dbl[][])  [unwired: 8 in, 1 out]
                  n181 = To Long Integer(number=w490) -> (32bit integer=w489:i32[][])
                  n182 = call-generic <vilib>:"NIMS_Get Scalar_w Error.vi"("A"=w489) -> ("Error Enum"=w473:T1, "Scalar"=w492:i32)  [unwired: 8 in, 1 out]
                  n183 = call-generic <vilib>:"NIMS_Complex To Real.vi"("A"=w494) -> ("Error Enum"=w476:T1, "Real(A)"=w493:dbl[][])  [unwired: 8 in, 1 out]
                  n184 = call-generic <vilib>:"NIMS_Get Scalar_w Error.vi"("A"=w493) -> ("Error Enum"=w475:T1, "Scalar"=w495:dbl)  [unwired: 8 in, 1 out]
                  n185 = call-generic <vilib>:"NIMS_Complex To Real.vi"("A"=w497) -> ("Error Enum"=w478:T1, "Real(A)"=w496:dbl[][])  [unwired: 8 in, 1 out]
                  n186 = call-generic <vilib>:"NIMS_Get Any Vector_w Error - Matrix.vi"("A"=w496) -> ("Error Enum"=w477:T1, "Vector"=w498:dbl[])  [unwired: 8 in, 1 out]
                  n187 = call-generic <vilib>:"NIMS_Complex To Real.vi"("A"=w500) -> ("Error Enum"=w480:T1, "Real(A)"=w499:dbl[][])  [unwired: 8 in, 1 out]
                  n188 = call-generic <vilib>:"NIMS_Get Any Vector_w Error - Matrix.vi"("A"=w499) -> ("Error Enum"=w479:T1, "Vector"=w501:dbl[])  [unwired: 8 in, 1 out]
                  n189 = call-generic <vilib>:"NIMS_Complex To Real.vi"("A"=w503) -> ("Error Enum"=w482:T1, "Real(A)"=w502:dbl[][])  [unwired: 8 in, 1 out]
                  n190 = call-generic <vilib>:"NIMS_Get Any Vector_w Error - Matrix.vi"("A"=w502) -> ("Error Enum"=w481:T1, "Vector"=w504:dbl[])  [unwired: 8 in, 1 out]
                  n191 = call-generic <vilib>:"NIMS_Complex To Real.vi"("A"=w506) -> ("Error Enum"=w484:T1, "Real(A)"=w505:dbl[][])  [unwired: 8 in, 1 out]
                  n192 = call-generic <vilib>:"NIMS_Get Any Vector_w Error - Matrix.vi"("A"=w505) -> ("Error Enum"=w483:T1, "Vector"=w507:dbl[])  [unwired: 8 in, 1 out]
                  n193 = call-generic <vilib>:"NIMS_Complex To Real.vi"("A"=w510) -> ("Error Enum"=w486:T1, "Real(A)"=w509:dbl[][])  [unwired: 8 in, 1 out]
                  n194 = To Long Integer(number=w509) -> (32bit integer=w508:i32[][])
                  n195 = call-generic <vilib>:"NIMS_Get Scalar_w Error.vi"("A"=w508) -> ("Error Enum"=w485:T1, "Scalar"=w511:i32)  [unwired: 8 in, 1 out]
                  n196 = call-generic <vilib>:"NIMS_Complex To Real.vi"("A"=w514) -> ("Error Enum"=w488:T1, "Real(A)"=w513:dbl[][])  [unwired: 8 in, 1 out]
                  n197 = To Long Integer(number=w513) -> (32bit integer=w512:i32[][])
                  n198 = call-generic <vilib>:"NIMS_Get Scalar_w Error.vi"("A"=w512) -> ("Error Enum"=w487:T1, "Scalar"=w515:i32)  [unwired: 8 in, 1 out]
                  n199 = call <vilib>:"NIMS_DF_iir_lpnormconstr.vi"("n"=w515, "e"=w504, "w"=w498, "p"=w492, "d"=w511, "f"=w507, "mag"=w501, "r"=w495) -> ("b"=w463:dbl[], "a"=w462:dbl[], "err"=w461:dbl, "SOS"=w460:dbl[][], "error"=w472:i32, "gain"=w459:dbl)  [unwired: 2 in]
                  n200 = Build Array(w466, w466, w466, w466, w466, w466, w466, w466, w466, w466, w466, w466, w466, w466, w466, w466, "iir_lpnormconstr") -> (w469:string[])
                  n201 = Build Array(w488, w487, w486, w485, w484, w483, w482, w481, w480, w479, w478, w477, w476, w475, w474, w473, w472) -> (w470:i32[])
                  n202 = call <vilib>:"NIMS_Create Error From Enums.vi"("Error Code"=bool[] [FALSE, FALSE, FALSE, FALSE, FALSE, FALSE, FALSE, FALSE, FALSE, FALSE, FALSE, FALSE, FALSE, FALSE, FALSE, FALSE, TRUE], "error in (no error)"=w468, "Line no"=w471, "Error Enums"=w470, "Function names"=w469) -> ("error out"=w464:errorcluster)  [unwired: 6 in]
                }
              }
              n203 = To Double Precision Complex(1:w403) -> (0:w402:cdb[][])
              n204 = call-generic <vilib>:"NIMS_RunTimeType_From StrictType (excl LVString).vi"("Plug-In Name"="", "Data In"=w402) -> ("Data Out"=w392:variant)  [unwired: 2 in]
              n205 = Initialize Array(w400, w399, w399) -> (w398:dbl[][])
              n206 = To Double Precision Complex(1:w398) -> (0:w397:cdb[][])
              n207 = call-generic <vilib>:"NIMS_RunTimeType_From StrictType (excl LVString).vi"("Plug-In Name"="", "Data In"=w397) -> ("Data Out"=w391:variant)  [unwired: 2 in]
              n208 = Initialize Array(w408, w407, w407) -> (w406:dbl[][])
              n209 = To Double Precision Complex(1:w406) -> (0:w405:cdb[][])
              n210 = call-generic <vilib>:"NIMS_RunTimeType_From StrictType (excl LVString).vi"("Plug-In Name"="", "Data In"=w405) -> ("Data Out"=w393:variant)  [unwired: 2 in]
              n211 = Build Array(w412) -> (w411:dbl[][])
              n212 = To Double Precision Complex(1:w411) -> (0:w410:cdb[][])
              n213 = call-generic <vilib>:"NIMS_RunTimeType_From StrictType (excl LVString).vi"("Plug-In Name"="", "Data In"=w410) -> ("Data Out"=w394:variant)  [unwired: 2 in]
              n214 = Build Array(w416) -> (w415:dbl[][])
              n215 = To Double Precision Complex(1:w415) -> (0:w414:cdb[][])
              n216 = call-generic <vilib>:"NIMS_RunTimeType_From StrictType (excl LVString).vi"("Plug-In Name"="", "Data In"=w414) -> ("Data Out"=w395:variant)  [unwired: 2 in]
              n217 = Build Array(w395, w394, w393, w392, w391) -> (w390:variant[])
            }
          }
        }
      }
    }
    frame Error {
    }
  }
  "error out" <- w3
  "[funct(A)]" <- w4
